vi "判断企业或用户归属地.vi"(8 "登录密码":string=" ", 9 "待查询用户名/手机号/邮箱":string=" ", 10 "待查询企业名":string=" ", 11 "个人剂量仪-云服务器.i":refnum<class "个人剂量仪-云服务器.lvclass">) -> (3 "账号密码通过？":bool)   [LabVIEW 2013, in "个人剂量仪-云服务器.lvclass"]
uses:
  <vilib>/addons/database/Connection.llb/Conn Execute.vi
  <vilib>/addons/database/NI_Database_API.lvlib
panel:
  out "所有企业名":string[](array[string])
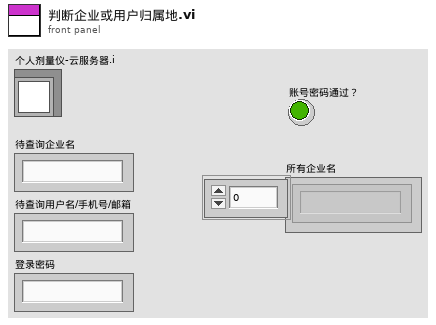
[diagram p1: front panel]
types:
  T1 = typedef "NI_Database_API.lvlib/Conn ObjectReference.ctl" = refnum<k1>
  T2 = cluster{"登录名":string, "密码":string, "企业名称":string, "邮箱":string, "电话":string}
  T3 = enum16{"用户名", "设备MAC", "设备状态", "密码", "职类", "姓名", "电话", "邮箱", "备注", "最后活动"}
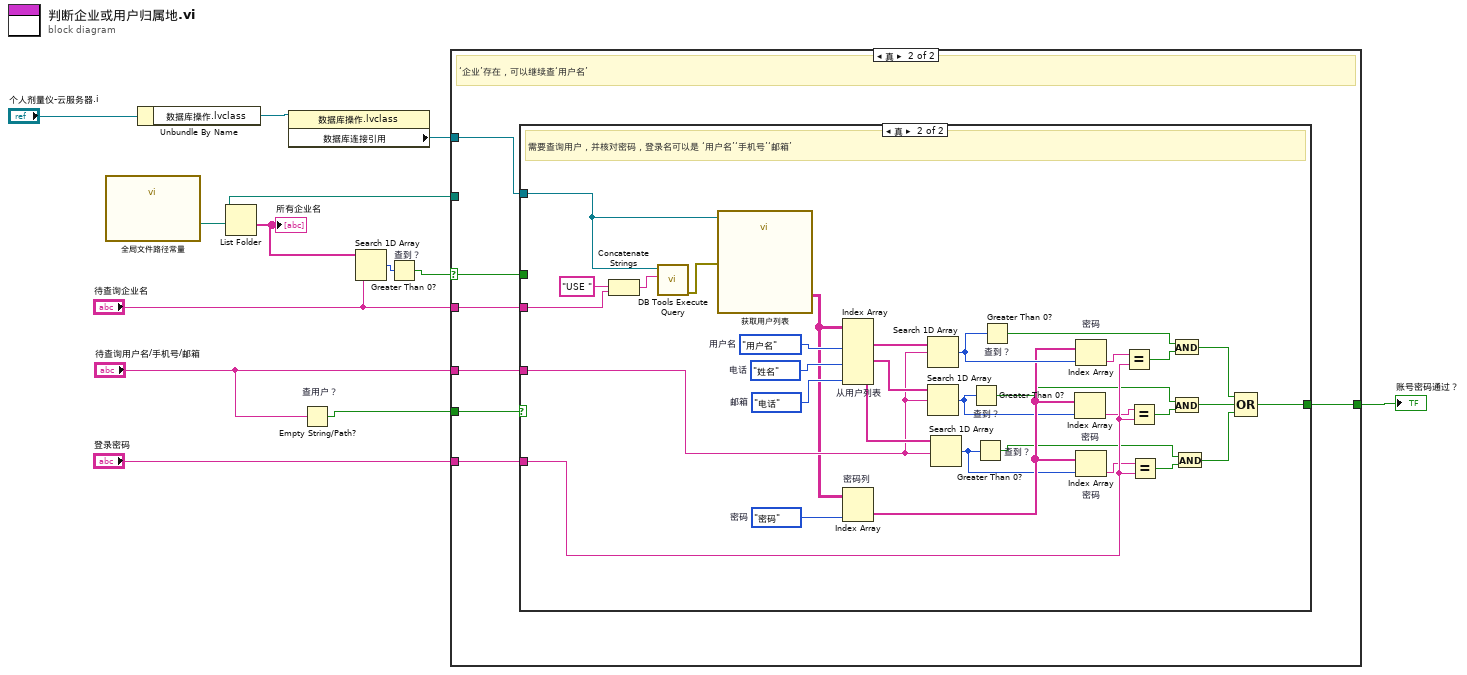
[diagram p0: block diagram]
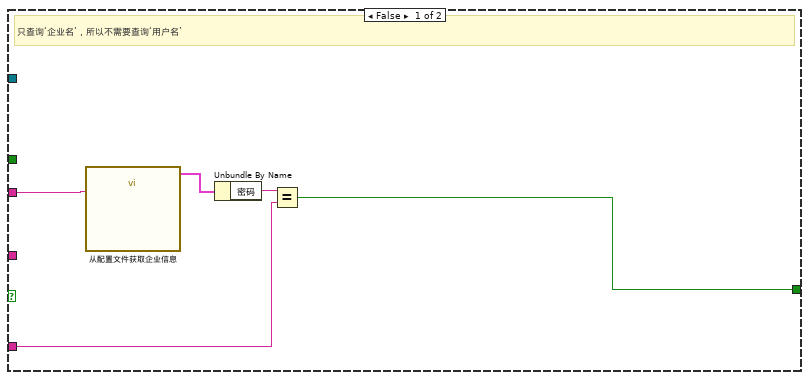
[diagram p3: hidden frame]
diagram:
  n1 = call "全局文件路径常量.vi"() -> ("用户数据库根目录"=w3:path)  [unwired: 9 in, 2 out]
  n2 = Unbundle By Name("个人剂量仪-云服务器.i") -> ("数据库操作.lvclass"=w12:refnum<class "数据库操作.lvclass">)
  n3 = List Folder(path=w3) -> (folder names=w10:string[])  [unwired: 3 in, 3 out]
  "所有企业名" <- w10
  n4 = property class="数据库操作.lvclass"(reference=w12) -> ("数据库连接引用"=w8:T1)  [unwired: 1 in, 2 out]
  n5 = Empty String/Path? "查用户？"(string/path="待查询用户名/手机号/邮箱") -> (empty?=w1:bool)
  n6 = Search 1D Array(1D array=w10, element="待查询企业名") -> (index of element=w9:i32)  [unwired: 1 in]
  n7 = Greater Than 0? "查到？"(x=w9) -> (x > 0?=w6:bool)
  n8 = case shown="真" w6 {
    selector: w6 -> [w13 w15]
    tunnel: w8 -> [_ w20]
    tunnel: "待查询企业名" -> [_ w19]
    tunnel: "待查询用户名/手机号/邮箱" -> [_ w18]
    tunnel: "登录密码" -> [_ w17]
    tunnel: [w13 w16] -> w4
    tunnel: w3 -> [_ _]
    tunnel: w1 -> [_ w14]
    frame False {
      # "‘企业’不存在，不需要继续查"
    }
    frame True {
      # "‘企业’存在，可以继续查‘用户名’"
      n9 = case shown="真" w14 {
        tunnel: w20 -> [_ w54]
        tunnel: w19 -> [w25 w56]
        tunnel: w18 -> [_ w46]
        tunnel: w17 -> [w22 w39]
        tunnel: [w21 w26] -> w16
        tunnel: w15 -> [_ _]
        frame False {
          # "只查询‘企业名’，所以不需要查询‘用户名’"
          n10 = call "从配置文件获取企业信息.vi"("登录名"=w25) -> ("企业信息"=w24:T2)  [unwired: 9 in, 1 out]
          n11 = Unbundle By Name(w24) -> ("密码"=w23:string)
          n12 = Equal?(x=w23, y=w22) -> (x = y?=w21:bool)
        }
        frame True {
          w44 = T3."密码"  # 密码
          w50 = T3."电话"  # 邮箱
          w51 = T3."姓名"  # 电话
          w52 = T3."用户名"  # 用户名
          # "需要查询用户，并核对密码，登录名可以是 ‘用户名’‘手机号’‘邮箱’"
          n13 = Concatenate Strings("USE ", w56) -> (w55:string)
          n14 = call-poly <vilib>:"DB Tools Execute Query.vi"("SQL query"=w55, "connection reference"=w54) -> ("error out"=w53:errorcluster)  [unwired: 6 in, 1 out]
          n15 = call "获取用户列表.vi"("error in (no error)"=w53, "数据库连接引用"=w54) -> ("用户列表"=w45:string[][])  [unwired: 4 in, 5 out]
          n16 = Index Array "从用户列表"(array=w45, index (col) #1=w52, index (col) #2=w51, index (col) #3=w50) -> (element #1=w49:string[], element #2=w48:string[], element #3=w47:string[])  [unwired: 3 in]
          n17 = Index Array "密码列"(array=w45, index (col)=w44) -> (element=w42:string[])  [unwired: 1 in]
          n18 = Search 1D Array(1D array=w49, element=w46) -> (index of element=w43:i32)  [unwired: 1 in]
          n19 = Search 1D Array(1D array=w48, element=w46) -> (index of element=w41:i32)  [unwired: 1 in]
          n20 = Search 1D Array(1D array=w47, element=w46) -> (index of element=w40:i32)  [unwired: 1 in]
          n21 = Greater Than 0? "查到？"(x=w41) -> (x > 0?=w32:bool)
          n22 = Greater Than 0? "查到？"(x=w40) -> (x > 0?=w30:bool)
          n23 = Greater Than 0? "查到？"(x=w43) -> (x > 0?=w34:bool)
          n24 = Index Array "密码"(array=w42, index=w41) -> (element=w37:string)
          n25 = Index Array "密码"(array=w42, index=w43) -> (element=w38:string)
          n26 = Index Array "密码"(array=w42, index=w40) -> (element=w36:string)
          n27 = Equal?(x=w38, y=w39) -> (x = y?=w35:bool)
          n28 = Equal?(x=w37, y=w39) -> (x = y?=w33:bool)
          n29 = Equal?(x=w36, y=w39) -> (x = y?=w31:bool)
          n30 = And(x=w34, y=w35) -> (x .and. y?=w29:bool)
          n31 = And(x=w32, y=w33) -> (x .and. y?=w28:bool)
          n32 = And(x=w30, y=w31) -> (x .and. y?=w27:bool)
          n33 = Compound Arithmetic op=OR(w29, w28, w27) -> (w26:bool)
        }
      }
    }
  }
  "账号密码通过？" <- w4
